vi "UI_Thread.vi"(10 "Event Registration Refnum":refnum<event-registration>, 11 "controller queue out":refnum<queue>) -> ()   [LabVIEW 2020]
uses:
  Controller_Response.ctl
  Controller_Response_Command.ctl
  Controller_Request.ctl
  Controller_Request_Command.ctl
  Main_Data.ctl
  BLE_Data_TargetDevice.ctl
  Main_Data_ACQ.ctl
  BLE_Data_Packet.ctl
panel:
  in  "Tab Control":enum32{"Page 1", "Page 2"}(tab)
  out "Notifications":bool
  out "Connected":bool
  in  "Scan_btn":bool
  in  "Stop_btn":bool
  in  "Target Address":string
  in  "Connection_btn":bool
  in  "Notifications_btn":bool
  out "Discovered devices":string[](array[string])
  out "Temperature":sgl[](graph)
  out "Acceleration":i16[][](graph)
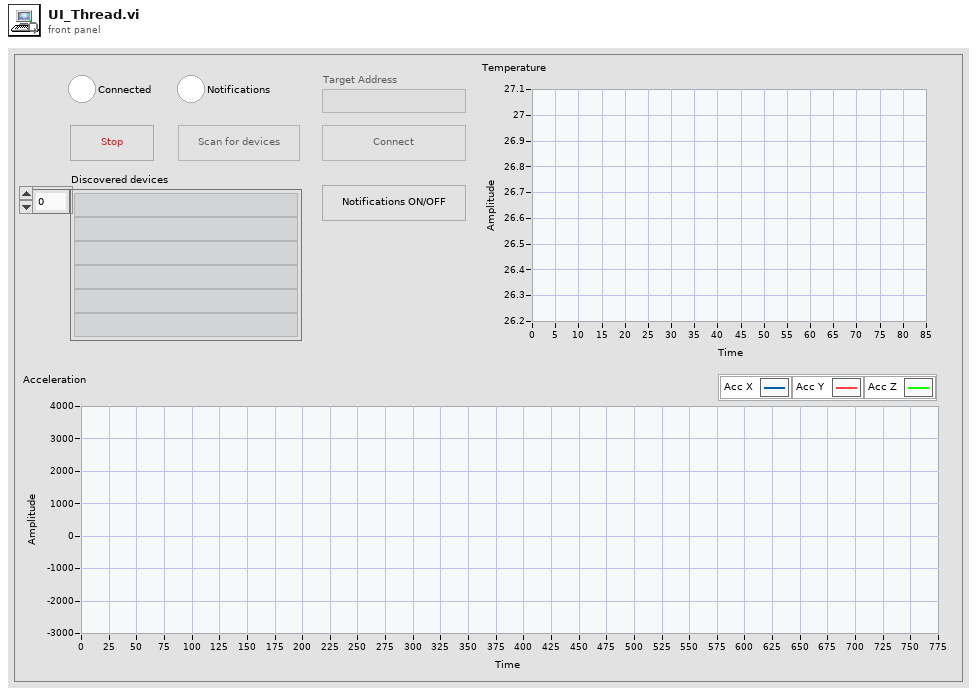
[diagram p1: front panel]
types:
  T1 = typedef "Main_Data.ctl" = cluster{"Scanned Devices":string[], "Target Device":T2, "ACQ Data":T3}
  T2 = typedef "BLE_Data_TargetDevice.ctl" = cluster{"IsConnected":bool, "Address":u64, "Notifications?":bool}
  T3 = typedef "Main_Data_ACQ.ctl" = cluster{"Temperature":sgl[], "Acceleration X":i16[], "Acceleration Y":i16[], "Acceleration Z":i16[]}
  T4 = enum8{"Enabled", "Disabled", "Disabled and Grayed Out"}
  T5 = typedef "Controller_Request.ctl" = cluster{"Command":T6, "Parameter":variant}
  T6 = typedef "Controller_Request_Command.ctl" = enum16{"BLE_ScannedDevices", "BLE_ConnectionResult", "BLE_NotificationToogleResult", "BLE_NotificationData", "BLE_ConnTimeout", "BLE_CloseResult", "User_Init", "User_ScanRequest", "User_ConnectionRequest", "User_CloseRequest", "User_NotficationToggleRequest"}
  T7 = typedef "Controller_Response_Command.ctl" = enum16{"Init", "ScanResult", "ConnectionResult", "ConnectionTimeout", "NotificationToogleResult", "NotificationData", "CloseResult"}
  T8 = cluster{"[0]":bool, "[1]":bool, "[2]":bool, "[3]":bool}
  T9 = typedef "BLE_Data_Packet.ctl" = cluster{"Temperature":cluster{"Available":bool, "Value":sgl}, "Acceleration X":cluster{"Available":bool, "Value":i16}, "Acceleration Y":cluster{"Available":bool, "Value":i16}, "Acceleration Z":cluster{"Available":bool, "Value":i16}}
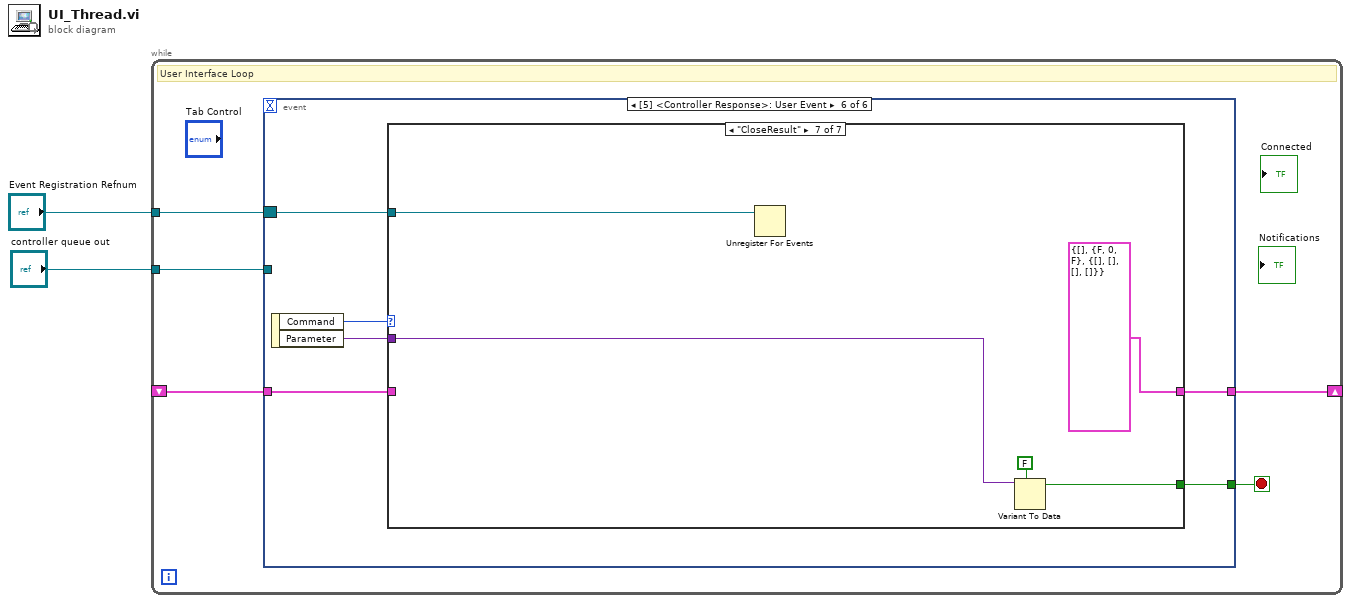
[diagram p0: block diagram]
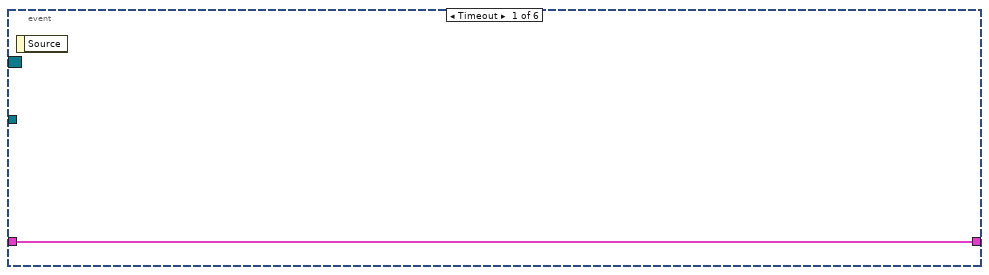
[diagram p2: hidden frame]
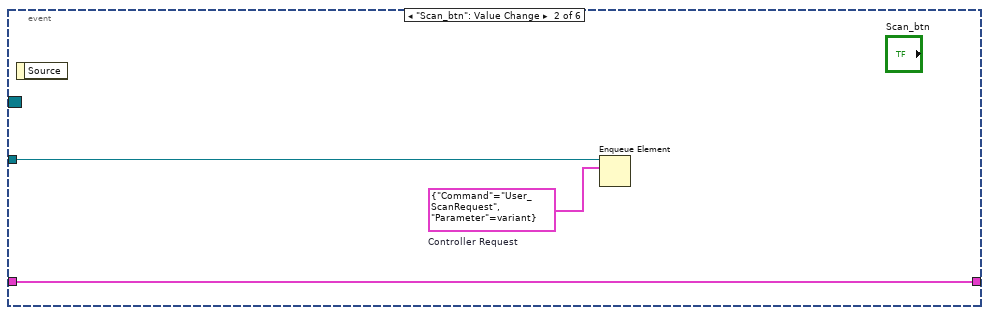
[diagram p3: hidden frame]
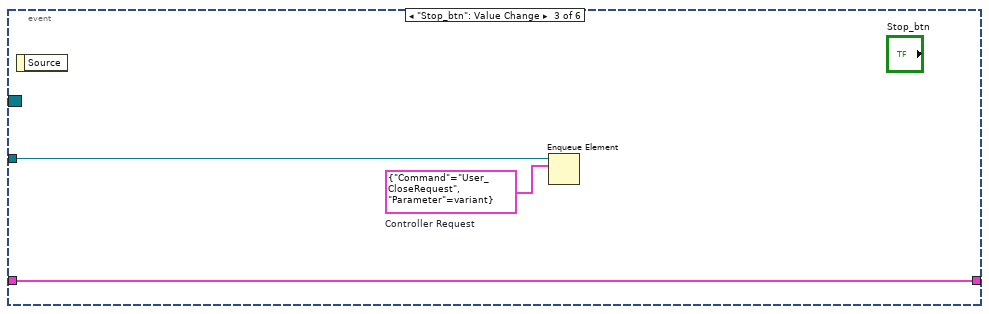
[diagram p4: hidden frame]
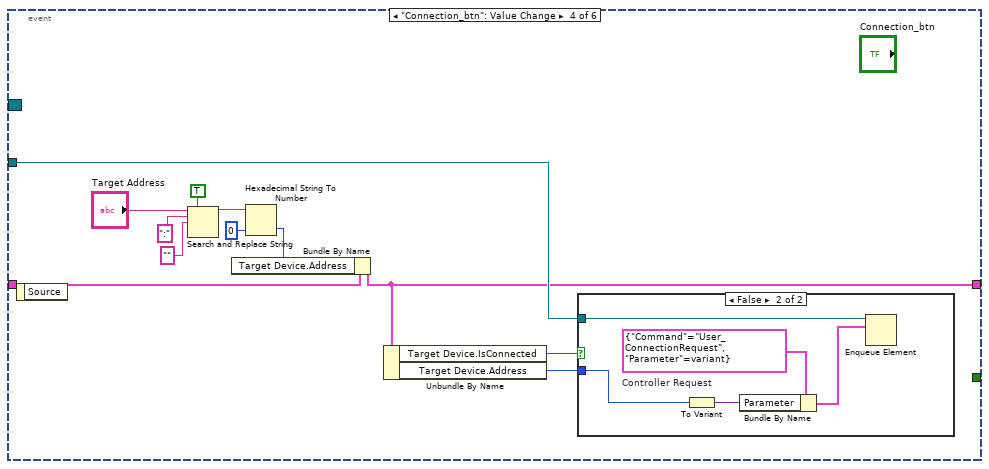
[diagram p5: hidden frame]
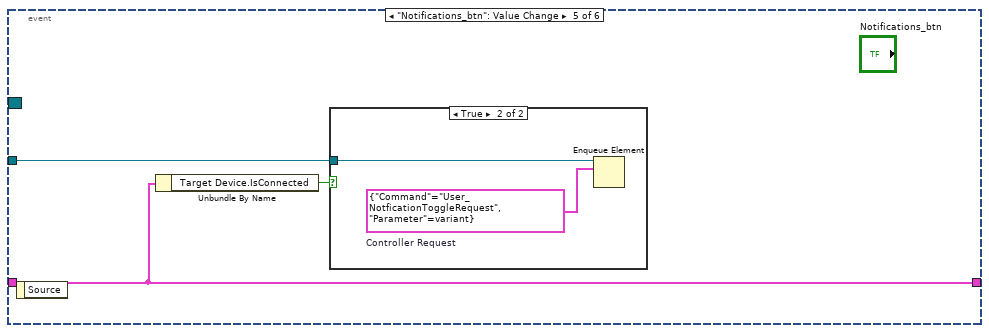
[diagram p7: hidden frame]
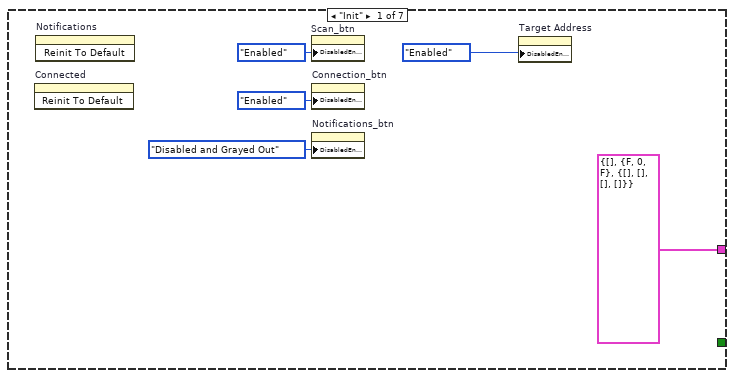
[diagram p9: hidden frame]
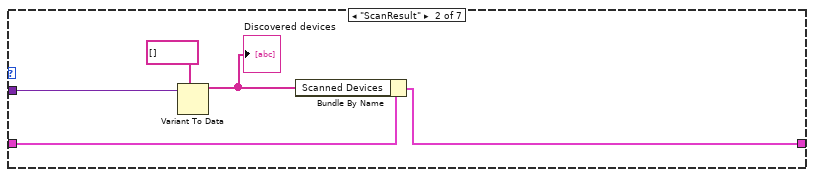
[diagram p10: hidden frame]
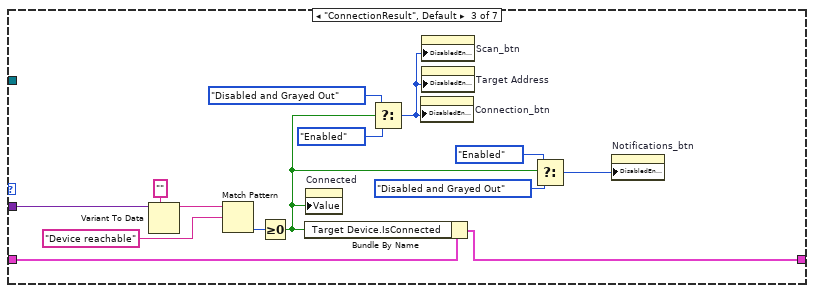
[diagram p11: hidden frame]
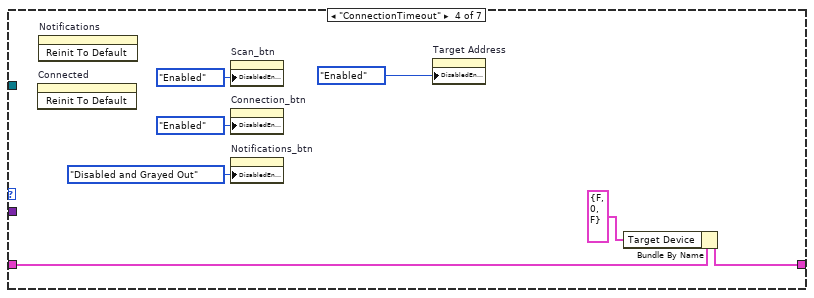
[diagram p12: hidden frame]
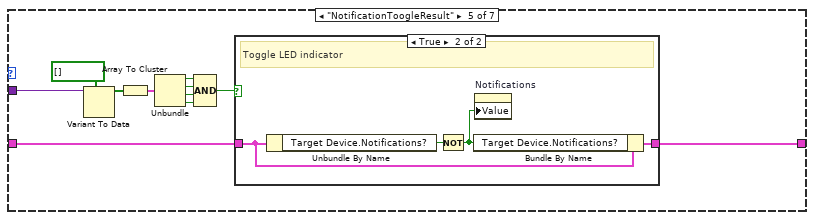
[diagram p13: hidden frame]
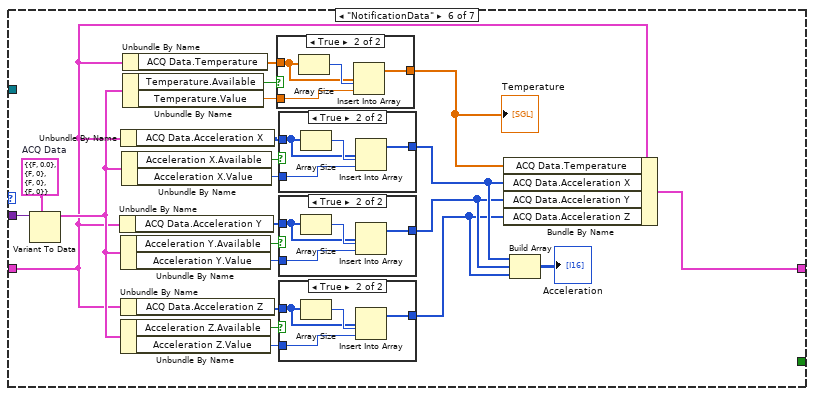
[diagram p15: hidden frame]
diagram:
  n1 = while {
    tunnel: "Event Registration Refnum" -> [w6]
    shift-right: [w5] -> _
    shift-left: _ -> [w4]
    tunnel: "controller queue out" -> [w3]
    stop <- w7 stop-if-true
    # "User Interface Loop"
    n2 = event shown="[5] <Controller Response>: User Event" {
      selector: w6 -> [_ _ _ _ _ w37]
      dyn-events: _ -> [_ _ _ _ _ _]
      timeout: _ -> [_ _ _ _ _ _]
      tunnel: [_ _ _ _ _ w38] -> w7
      tunnel: w3 -> [_ w9 w12 w18 w34 _]
      tunnel: [w8 w11 w14 w16 w32 w39] -> w5
      tunnel: w4 -> [w8 w11 w14 w20 w32 w40]
      event Timeout {
        n3 = event-data() -> ()  [unwired: 1 in, 1 out]
      }
      event "Scan_btn": Value Change {
        w10 = T5 {"Command"=enum."User_ScanRequest", "Parameter"=variant}  # Controller Request
        n4 = event-data() -> ()  [unwired: 1 in, 1 out]
        n5 = Enqueue Element(queue=w9, element=w10) -> ()  [unwired: 2 in, 3 out]
      }
      event "Stop_btn": Value Change {
        w13 = T5 {"Command"=enum."User_CloseRequest", "Parameter"=variant}  # Controller Request
        n6 = event-data() -> ()  [unwired: 1 in, 1 out]
        n7 = Enqueue Element(queue=w12, element=w13) -> ()  [unwired: 2 in, 3 out]
      }
      event "Connection_btn": Value Change {
        n8 = event-data() -> ()  [unwired: 1 in, 1 out]
        n9 = Search and Replace String(replace all?=TRUE ("replace all? (F)"), input string="Target Address", search string=":", replace string="" ("replace string (\"\")")) -> (result string=w23:string)  [unwired: 4 in, 3 out]
        n10 = Hexadecimal String To Number(string=w23, default (0uL)=u64 0 ("default (0 U32)")) -> (number=w21:u64)  [unwired: 1 in, 1 out]
        n11 = Bundle By Name(cluster=w20, "Target Device.Address"=w21) -> (w16:T1)
        n12 = Unbundle By Name(w16) -> ("Target Device.IsConnected"=w19:bool, "Target Device.Address"=w17:u64)
        n13 = case shown="False" w19 {
          tunnel: w18 -> [_ w31]
          tunnel: w17 -> [_ w29]
          frame True {
          }
          frame False {
            w28 = T5 {"Command"=enum."User_ConnectionRequest", "Parameter"=variant}  # Controller Request
            n14 = To Variant(anything=w29) -> (Variant=w30:variant)
            n15 = Bundle By Name(cluster=w28, "Parameter"=w30) -> (w27:T5)
            n16 = Enqueue Element(queue=w31, element=w27) -> ()  [unwired: 2 in, 3 out]
          }
        }
      }
      event "Notifications_btn": Value Change {
        n17 = event-data() -> ()  [unwired: 1 in, 1 out]
        n18 = Unbundle By Name(w32) -> ("Target Device.IsConnected"=w33:bool)
        n19 = case shown="True" w33 {
          tunnel: w34 -> [_ w36]
          frame False {
          }
          frame True {
            w35 = T5 {"Command"=enum."User_NotficationToggleRequest", "Parameter"=variant}  # Controller Request
            n20 = Enqueue Element(queue=w36, element=w35) -> ()  [unwired: 2 in, 3 out]
          }
        }
      }
      event User Event {
        n21 = event-data() -> ("Command"=w42:T7, "Parameter"=w41:variant)  [unwired: 1 in]
        n22 = case shown="\"CloseResult\"" w42 {
          tunnel: w41 -> [_ w51 w61 _ w83 w111 w134]
          tunnel: w40 -> [_ w50 w62 w69 w82 w102 _]
          tunnel: [T1 {"Scanned Devices"=[], "Target Device"={"IsConnected"=FALSE, "Address"=0, "Notifications?"=FALSE}, "ACQ Data"={"Temperature"=[], "Acceleration X"=[], "Acceleration Y"=[], "Acceleration Z"=[]}} w49 w58 w68 w81 w108 T1 {"Scanned Devices"=[], "Target Device"={"IsConnected"=FALSE, "Address"=0, "Notifications?"=FALSE}, "ACQ Data"={"Temperature"=[], "Acceleration X"=[], "Acceleration Y"=[], "Acceleration Z"=[]}}] -> w39
          tunnel: [_ _ _ _ _ _ w135] -> w38
          tunnel: w37 -> [_ _ _ _ _ _ w132]
          frame "Init" {
            n23 = invoke on="Connected" class="Bool (strict)" method="Reinit To Default"() -> ()  [unwired: 3 in, 3 out]
            n24 = invoke on="Notifications" class="Bool (strict)" method="Reinit To Default"() -> ()  [unwired: 3 in, 3 out]
            n25 = property on="Scan_btn" class="Bool"("DisabledEnum"=T4."Enabled" ("Disabled")) -> ()  [unwired: 2 in, 2 out]
            n26 = property on="Connection_btn" class="Bool"("DisabledEnum"=T4."Enabled" ("Disabled")) -> ()  [unwired: 2 in, 2 out]
            n27 = property on="Notifications_btn" class="Bool"("DisabledEnum"=T4."Disabled and Grayed Out" ("Disabled")) -> ()  [unwired: 2 in, 2 out]
            n28 = property on="Target Address" class="Str"("DisabledEnum"=T4."Enabled" ("Disabled")) -> ()  [unwired: 2 in, 2 out]
          }
          frame "ScanResult" {
            n29 = Variant To Data(type=string[] [], Variant=w51) -> (data=w48:string[])  [unwired: 1 in, 1 out]
            "Discovered devices" <- w48
            n30 = Bundle By Name(cluster=w50, "Scanned Devices"=w48) -> (w49:T1)
          }
          frame "ConnectionResult", Default {
            n31 = Variant To Data(type="", Variant=w61) -> (data=w65:string)  [unwired: 1 in, 1 out]
            n32 = Match Pattern(string=w65, regular expression="Device reachable") -> (offset past match=w66:i32)  [unwired: 1 in, 3 out]
            n33 = Greater Or Equal To 0?(x=w66) -> (x >= 0?=w55:bool)
            n34 = Bundle By Name(cluster=w62, "Target Device.IsConnected"=w55) -> (w58:T1)
            n35 = property on="Connected" class="Bool (strict)"("Value"=w55) -> ()  [unwired: 2 in, 2 out]
            n36 = Select(t=T4."Disabled and Grayed Out" ("Disabled"), s=w55, f=T4."Enabled") -> (s? t:f=w53:T4)
            n37 = property on="Connection_btn" class="Bool"("DisabledEnum"=w53) -> ()  [unwired: 2 in, 2 out]
            n38 = property on="Scan_btn" class="Bool"("DisabledEnum"=w53) -> ()  [unwired: 2 in, 2 out]
            n39 = property on="Target Address" class="Str"("DisabledEnum"=w53) -> ()  [unwired: 2 in, 2 out]
            n40 = Select(t=T4."Enabled" ("Disabled"), s=w55, f=T4."Disabled and Grayed Out") -> (s? t:f=w54:T4)
            n41 = property on="Notifications_btn" class="Bool"("DisabledEnum"=w54) -> ()  [unwired: 2 in, 2 out]
          }
          frame "ConnectionTimeout" {
            n42 = invoke on="Connected" class="Bool (strict)" method="Reinit To Default"() -> ()  [unwired: 3 in, 3 out]
            n43 = invoke on="Notifications" class="Bool (strict)" method="Reinit To Default"() -> ()  [unwired: 3 in, 3 out]
            n44 = property on="Scan_btn" class="Bool"("DisabledEnum"=T4."Enabled" ("Disabled")) -> ()  [unwired: 2 in, 2 out]
            n45 = property on="Connection_btn" class="Bool"("DisabledEnum"=T4."Enabled" ("Disabled")) -> ()  [unwired: 2 in, 2 out]
            n46 = property on="Notifications_btn" class="Bool"("DisabledEnum"=T4."Disabled and Grayed Out" ("Disabled")) -> ()  [unwired: 2 in, 2 out]
            n47 = property on="Target Address" class="Str"("DisabledEnum"=T4."Enabled" ("Disabled")) -> ()  [unwired: 2 in, 2 out]
            n48 = Bundle By Name(cluster=w69, "Target Device"=T2 {"IsConnected"=FALSE, "Address"=0, "Notifications?"=FALSE}) -> (w68:T1)
          }
          frame "NotificationToogleResult" {
            n49 = Variant To Data(type=bool[] [], Variant=w83) -> (data=w80:bool[])  [unwired: 1 in, 1 out]
            n50 = Array To Cluster(array=w80) -> (cluster=w79:T8)
            n51 = Unbundle(w79) -> ("[0]"=w78:bool, "[1]"=w77:bool, "[2]"=w76:bool, "[3]"=w75:bool)
            n52 = Compound Arithmetic op=AND(w78, w77, w76, w75) -> (w74:bool)
            n53 = case shown="True" w74 {
              tunnel: w82 -> [w85 w89]
              tunnel: [w85 w87] -> w81
              frame False {
              }
              frame True {
                # "Toggle LED indicator"
                n54 = Unbundle By Name(w89) -> ("Target Device.Notifications?"=w88:bool)
                n55 = Not(x=w88) -> (.not. x?=w86:bool)
                n56 = Bundle By Name(cluster=w89, "Target Device.Notifications?"=w86) -> (w87:T1)
                n57 = property on="Notifications" class="Bool (strict)"("Value"=w86) -> ()  [unwired: 2 in, 2 out]
              }
            }
          }
          frame "NotificationData" {
            w110 = T9 {"Temperature"={"Available"=FALSE, "Value"=0.0}, "Acceleration X"={"Available"=FALSE, "Value"=0}, "Acceleration Y"={"Available"=FALSE, "Value"=0}, "Acceleration Z"={"Available"=FALSE, "Value"=0}}  # ACQ Data
            n58 = Variant To Data(type=w110, Variant=w111) -> (data=w109:T9)  [unwired: 1 in, 1 out]
            n59 = Unbundle By Name(w102) -> ("ACQ Data.Acceleration Y"=w98:i16[])
            n60 = Unbundle By Name(w102) -> ("ACQ Data.Acceleration X"=w104:i16[])
            n61 = Unbundle By Name(w109) -> ("Acceleration Y.Available"=w97:bool, "Acceleration Y.Value"=w96:i16)
            n62 = Unbundle By Name(w102) -> ("ACQ Data.Acceleration Z"=w99:i16[])
            n63 = Unbundle By Name(w109) -> ("Acceleration Z.Available"=w100:bool, "Acceleration Z.Value"=w101:i16)
            n64 = Unbundle By Name(w109) -> ("Acceleration X.Available"=w90:bool, "Acceleration X.Value"=w103:i16)
            n65 = Unbundle By Name(w102) -> ("ACQ Data.Temperature"=w107:sgl[])
            n66 = Unbundle By Name(w109) -> ("Temperature.Available"=w106:bool, "Temperature.Value"=w105:sgl)
            n67 = case shown="True" w106 {
              tunnel: w107 -> [w127 w130]
              tunnel: w105 -> [_ w129]
              tunnel: [w127 w128] -> w95
              frame False {
              }
              frame True {
                n68 = Array Size(array=w130) -> (size(s)=w131:i32)
                n69 = Insert Into Array(array=w130, index=w131, new element=w129) -> (w128:sgl[])
              }
            }
            "Temperature" <- w95
            n70 = case shown="True" w90 {
              tunnel: w104 -> [w122 w125]
              tunnel: w103 -> [_ w124]
              tunnel: [w122 w123] -> w94
              frame False {
              }
              frame True {
                n71 = Array Size(array=w125) -> (size(s)=w126:i32)
                n72 = Insert Into Array(array=w125, index=w126, new element=w124) -> (w123:i16[])
              }
            }
            n73 = case shown="True" w97 {
              tunnel: w98 -> [w117 w120]
              tunnel: w96 -> [_ w119]
              tunnel: [w117 w118] -> w93
              frame False {
              }
              frame True {
                n74 = Array Size(array=w120) -> (size(s)=w121:i32)
                n75 = Insert Into Array(array=w120, index=w121, new element=w119) -> (w118:i16[])
              }
            }
            n76 = case shown="True" w100 {
              tunnel: w99 -> [w112 w115]
              tunnel: w101 -> [_ w114]
              tunnel: [w112 w113] -> w92
              frame False {
              }
              frame True {
                n77 = Array Size(array=w115) -> (size(s)=w116:i32)
                n78 = Insert Into Array(array=w115, index=w116, new element=w114) -> (w113:i16[])
              }
            }
            n79 = Bundle By Name(cluster=w102, "ACQ Data.Temperature"=w95, "ACQ Data.Acceleration X"=w94, "ACQ Data.Acceleration Y"=w93, "ACQ Data.Acceleration Z"=w92) -> (w108:T1)
            n80 = Build Array(w94, w93, w92) -> (→"Acceleration":i16[][])
          }
          frame "CloseResult" {
            n81 = Unregister For Events(event registration refnum=w132) -> ()  [unwired: 1 in, 1 out]
            n82 = Variant To Data(type=FALSE, Variant=w134) -> (data=w135:bool)  [unwired: 1 in, 1 out]
          }
        }
      }
    }
  }
